vi "Process XML Node old.vi"(8 "Error in":errorcluster caption="Error in (no error)", 11 "XML Element":refnum<k20>) -> (0 "Error out":errorcluster, 1 "Is Array?":bool, 2 "Data Item":refnum<class "Data Item.lvclass">, 3 "XML Element Out":refnum<k20>)   [LabVIEW 2018]
uses:
  Data Item.lvclass
  Attribute.lvclass
  Data Item.lvclass/Data Item.ctl
  Attribute.lvclass/Attribute.ctl
  Element.lvclass/Element.ctl
  Element.lvclass
  C:/Users/Flarn/Documents/LabVIEW Projects/Low-Level VI Manipulation/Support Files/VILab/Data Item.lvclass
  Attribute/Create Attribute (String).vi
  Attribute/Create Attribute (Data Item).vi
  Data Item/Create Basic Data Item.vi
  Element Array.lvclass
  <vilib>/xml/NI_XML.lvlib
  <resource>/objmgr/DOMUserDefRef.rc
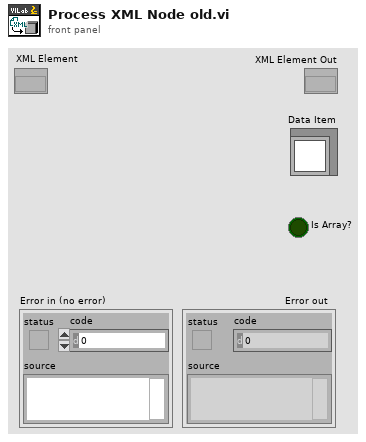
[diagram p1: front panel]
types:
  T1 = cluster{"class":string, "uid":string, "Attributes":refnum<class "Attribute.lvclass">[], "Array?":bool}
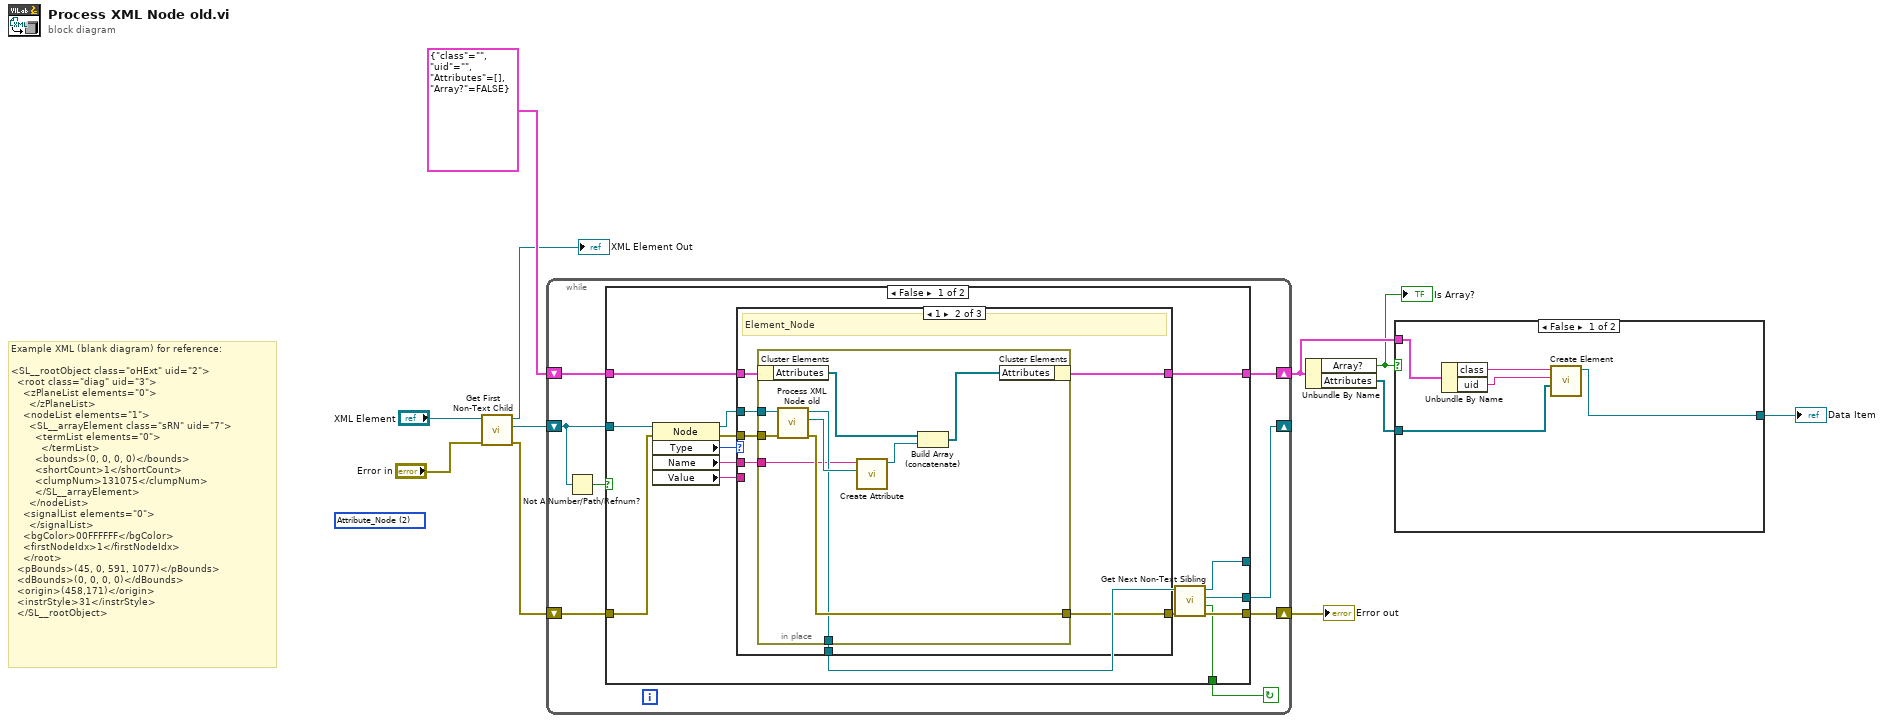
[diagram p0: block diagram]
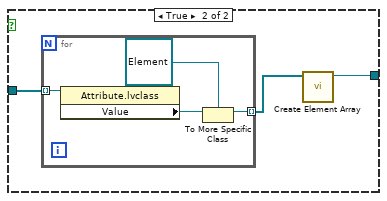
[diagram p2: hidden frame]
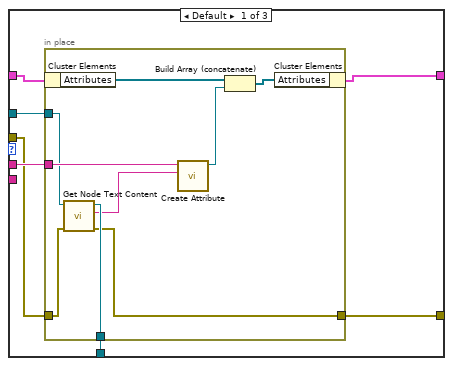
[diagram p3: hidden frame]
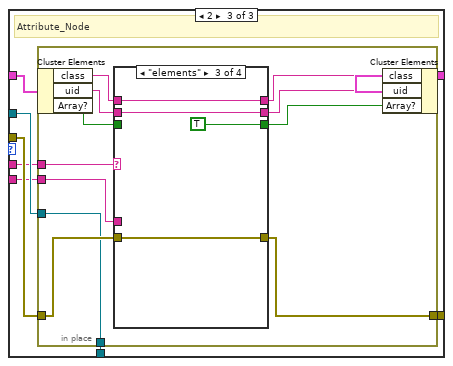
[diagram p4: hidden frame]
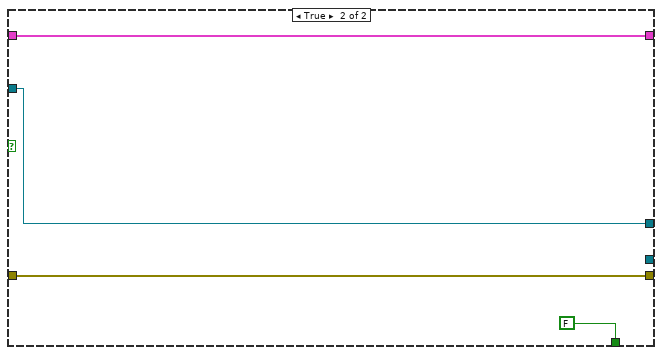
[diagram p8: hidden frame]
diagram:
  (unwired) 2 items=["Element_Node"=1, "Attribute_Node"=2, "Text_Node"=3, "CDATASection_Node"=4, "EntityReference_Node"=5, "Entity_Node"=6, "ProcessingInstruction_Node"=7, "Comment_Node"=8, "Document_Node"=9, "DocumentType_Node"=10, "DocumentFragment_Node"=11, "Notation_Node"=12] ("Node Type")
  # "Example XML (blank diagram) for reference:\n\n<SL__rootObject class=\"oHExt\" uid=\"2\">\n  <root class=\"diag\" uid=\"3\">\n    <zPlaneList elements=\"0\">\n      </zPlaneList>\n    <nodeList elements=\"1\">\n      <SL__arrayElement class=\"sRN\" uid=\"7\">\n        <termList elements=\"0\">\n          </termList>\n        <bounds>(0, 0, 0, 0)</bounds>\n        <shortCount>1</shortCount>\n        <clumpNum>131075</clumpNum>\n        </SL__arrayElement>\n      </nodeList>\n    <signalList elements=\"0\">\n      </signalList>\n    <bgColor>00FFFFFF</bgColor>\n    <firstNodeIdx>1</firstNodeIdx>\n    </root>\n  <pBounds>(45, 0, 591, 1077)</pBounds>\n  <dBounds>(0, 0, 0, 0)</dBounds>\n  <origin>(458,171)</origin>\n  <instrStyle>31</instrStyle>\n  </SL__rootObject>"
  n1 = call <vilib>:"Get First Non-Text Child.vi"("error in (no error)"="Error in", "node in"="XML Element") -> ("error out"=w8:errorcluster, "child node"=w10:refnum<k20>, "node out"=→"XML Element Out":refnum<k20>)  [unwired: 6 in, 1 out]
  n2 = while {
    shift-right: [w15] -> w3
    shift-left: T1 {"class"="", "uid"="", "Attributes"=[], "Array?"=FALSE} -> [w16]
    shift-right: [w19] -> w7
    shift-left: w8 -> [w17]
    shift-right: [w14] -> _
    shift-left: w10 -> [w12]
    stop <- w18 continue-if-true
    n3 = Not A Number/Path/Refnum?(number/path/refnum=w12) -> (NaN/Path/Refnum?=w13:bool)
    n4 = case shown="False" w13 {
      tunnel: [w34 w105] -> w19
      tunnel: [w33 FALSE ("found sibling node?")] -> w18
      tunnel: w12 -> [w32 w102]
      tunnel: w17 -> [w30 w105]
      tunnel: w16 -> [w27 w103]
      tunnel: [w26 w103] -> w15
      tunnel: [w24 _] -> w14
      tunnel: [w22 w102] -> _
      frame False {
        n5 = property class="Node"(reference=w32, error in=w30) -> (reference out=w28:refnum<k20>, error out=w29:errorcluster, "Type"=w31:i32, "Name"=w21:string, "Value"=w20:string)
        n6 = case shown="1" w31 {
          tunnel: w29 -> [w36 w57 w74]
          tunnel: w28 -> [w40 w56 w71]
          tunnel: w27 -> [w38 w55 w72]
          tunnel: [w37 w54 w73] -> w26
          tunnel: [w35 w53 w70] -> w25
          tunnel: [w41 w52 w69] -> w23
          tunnel: w21 -> [w39 w51 w68]
          tunnel: w20 -> [_ _ w67]
          frame Default {
            n7 = in-place {
              in-place-border: [w45] -> w41
              in-place-border: w40 -> [w46]
              in-place-border: w39 -> [w50]
              in-place-border: w36 -> [w44]
              in-place-border: [w43] -> w35
              n8 = in-place-cluster #1(w38) -> ("Attributes"=w49:refnum<class "Attribute.lvclass">[])
              n9 = call <vilib>:"Get Node Text Content.vi"("error in (no error)"=w44, "node in"=w46) -> ("error out"=w43:errorcluster, "node text"=w42:string, "node out"=w45:refnum<k20>)  [unwired: 7 in]
              n10 = call-poly "Create Attribute.vi"("Value"=w42, "Name"=w50) -> ("Attribute"=w48:refnum<class "Attribute.lvclass">)  [unwired: 9 in]
              n11 = Build Array (concatenate)(w49, w48) -> (w47:refnum<class "Attribute.lvclass">[])
              n12 = in-place-cluster #1("Attributes"=w47) -> (w37:T1)
            }
          }
          frame 1 {
            # "Element_Node"
            n13 = in-place {
              in-place-border: w57 -> [w66]
              in-place-border: w56 -> [w65]
              in-place-border: [w60] -> w53
              in-place-border: [w59] -> w52
              in-place-border: w51 -> [w58]
              n14 = in-place-cluster #2(w55) -> ("Attributes"=w62:refnum<class "Attribute.lvclass">[])
              n15 = call "Process XML Node old.vi"("Error in"=w66, "XML Element"=w65) -> ("Error out"=w60:errorcluster, "Data Item"=w64:refnum<class "Data Item.lvclass">, "XML Element Out"=w59:refnum<k20>)  [unwired: 6 in, 1 out]
              n16 = call-poly "Create Attribute.vi"("Value"=w64, "Name"=w58) -> ("Attribute"=w63:refnum<class "Attribute.lvclass">)  [unwired: 9 in]
              n17 = Build Array (concatenate)(w62, w63) -> (w61:refnum<class "Attribute.lvclass">[])
              n18 = in-place-cluster #2("Attributes"=w61) -> (w54:T1)
            }
          }
          frame 2 {
            # "Attribute_Node"
            n19 = in-place {
              in-place-border: w74 -> [w78]
              in-place-border: w68 -> [w85]
              in-place-border: w71 -> [w76]
              in-place-border: [w77] -> w70
              in-place-border: [w76] -> w69
              in-place-border: w67 -> [w75]
              n20 = in-place-cluster #3(w72) -> ("class"=w84:string, "uid"=w83:string, "Array?"=w82:bool)
              n21 = case shown="\"elements\"" w85 {
                tunnel: w84 -> [_ w93 w97 w101]
                tunnel: w83 -> [w89 _ w96 w100]
                tunnel: w82 -> [w88 w92 _ w99]
                tunnel: [w86 w93 w97 w101] -> w81
                tunnel: [w89 w90 w96 w100] -> w80
                tunnel: [w88 w92 TRUE w99] -> w79
                tunnel: w78 -> [w87 w91 w95 w98]
                tunnel: [w87 w91 w95 w98] -> w77
                tunnel: w75 -> [w86 w90 _ _]
                frame "class" {
                }
                frame "uid" {
                }
                frame "elements" {
                }
                frame Default {
                }
              }
              n22 = in-place-cluster #3("class"=w81, "uid"=w80, "Array?"=w79) -> (w73:T1)
            }
          }
        }
        n23 = call <vilib>:"Get Next Non-Text Sibling.vi"("error in (no error)"=w25, "node in"=w23) -> ("error out"=w34:errorcluster, "found sibling node?"=w33:bool, "sibling node"=w24:refnum<k20>, "node out"=w22:refnum<k20>)  [unwired: 6 in]
      }
      frame True {
      }
    }
  }
  "Error out" <- w7
  n24 = Unbundle By Name(w3) -> ("Array?"=w2:bool, "Attributes"=w5:refnum<class "Attribute.lvclass">[])
  "Is Array?" <- w2
  n25 = case shown="False" w2 {
    tunnel: w5 -> [w107 w113]
    tunnel: [w106 w111] -> w4
    tunnel: w3 -> [w110 _]
    frame False {
      n26 = Unbundle By Name(w110) -> ("class"=w109:string, "uid"=w108:string)
      n27 = call "Create Element.vi"("Attributes"=w107, "uid"=w108, "class"=w109) -> ("Element"=w106:refnum<class "Element.lvclass">)  [unwired: 8 in]
    }
    frame True {
      n28 = for {
        tunnel: w113 -> [w117] mode=indexing
        tunnel: [w114] -> w112 mode=indexing
        n29 = property class="Attribute.lvclass"(reference=w117) -> ("Value"=w116:refnum<class "Data Item.lvclass">)  [unwired: 1 in, 2 out]
        n30 = To More Specific Class(target class=refnum<class "Element.lvclass"> refnum ("VILab.lvlib:Element.lvclass"), reference=w116) -> (specific class reference=w114:refnum<class "Element.lvclass">)  [unwired: 1 in, 1 out]
      }
      n31 = call "Create Element Array.vi"("Contents"=w112) -> ("Element Array"=w111:refnum<class "Element Array.lvclass">)  [unwired: 9 in, 1 out]
    }
  }
  "Data Item" <- w4
